vi "Process File.vi"(8 "error in (no error)":errorcluster, 10 "File":path, 11 "NHMFL Synthesizer in":refnum<class "NHMFL Synthesizer.lvclass">) -> (0 "error out":errorcluster, 2 "File out":path, 3 "NHMFL Synthesizer out":refnum<class "NHMFL Synthesizer.lvclass">)   [LabVIEW 2016, in "NHMFL Synthesizer.lvclass"]
uses:
  NHMFL Synthesizer.lvclass
  NHMFL Synthesizer.lvclass/NHMFL Synthesizer.ctl
  Read NHMFL Synthesizer Configuration.vi
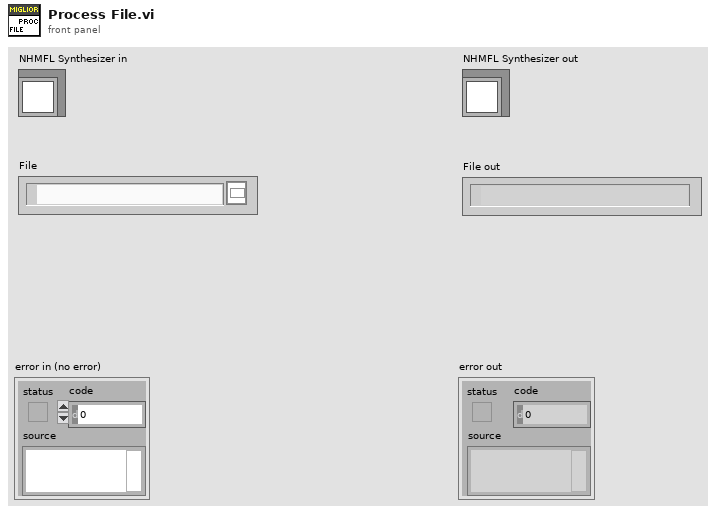
[diagram p1: front panel]
types:
  T1 = enum16{"open", "open or create", "create or replace", "create", "open (read-only)"}
  T2 = typedef "Actual Settings.ctl" = cluster{"Clock/F1":ext, "Clock/F2":ext, "F1":ext, "F2":ext, "Clock":ext}
  T3 = typedef "NHMFL Synthesizer Configuration.ctl" = cluster{"DAQmx Device":tag, "Variable amplitude frequency":dbl, "Fixed amplitude frequency":dbl, "Amplitude":dbl, "Clock multiplier":i32, "Cannel names (variable F)":string[], "Cannel names (fixed F)":string[], "Group":string}
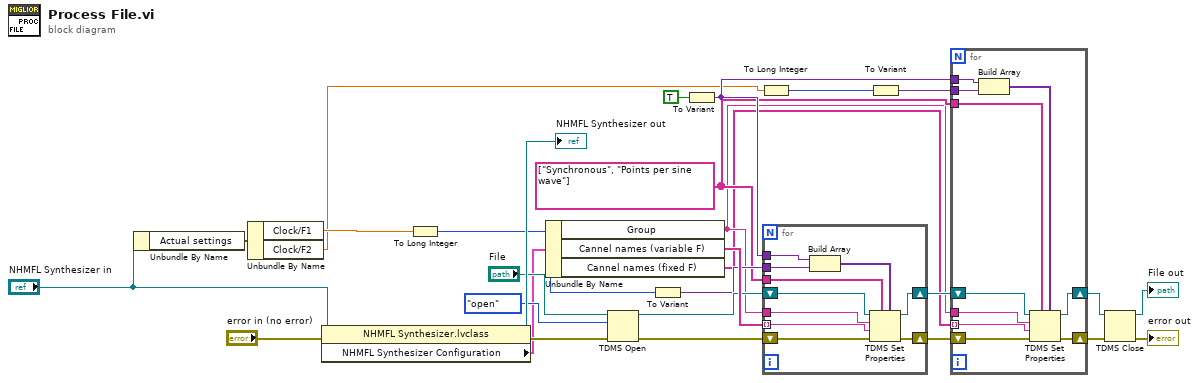
[diagram p0: block diagram]
diagram:
  w7 = string[] ["Synchronous", "Points per sine wave"] ("property names")
  n1 = Unbundle By Name("NHMFL Synthesizer in") -> ("Actual settings"=w18:T2)
  n2 = Unbundle By Name(w18) -> ("Clock/F1"=w16:ext, "Clock/F2"=w10:ext)
  n3 = property class="NHMFL Synthesizer.lvclass"(reference="NHMFL Synthesizer in", error in="error in (no error)") -> (reference out=→"NHMFL Synthesizer out":refnum<class "NHMFL Synthesizer.lvclass">, error out=w24:errorcluster, "NHMFL Synthesizer Configuration"=w22:T3)
  n4 = To Long Integer(number=w16) -> (32bit integer=w15:i32)
  n5 = Unbundle By Name(w22) -> ("Group"=w6:string, "Cannel names (variable F)"=w21:string[], "Cannel names (fixed F)"=w5:string[])
  n6 = TDMS Open(8:w24, 10:T1."open" ("operation (0:open)"), 11:"File") -> (0:w19:errorcluster, 3:w20:refnum<k34>)  [unwired: 4 in]
  n7 = To Variant(anything=w15) -> (Variant=w14:variant)
  n8 = To Variant(anything=TRUE) -> (Variant=w11:variant)
  n9 = To Long Integer(number=w10) -> (32bit integer=w9:i32)
  n10 = for {
    tunnel: w21 -> [w35] mode=indexing
    shift-right: [w33] -> w13
    shift-left: w20 -> [w38]
    shift-right: [w34] -> w12
    shift-left: w19 -> [w37]
    tunnel: w6 -> [w36]
    tunnel: w7 -> [w32]
    tunnel: w11 -> [w31]
    tunnel: w14 -> [w30]
    n11 = Build Array(w31, w30) -> (w29:variant[])
    n12 = TDMS Set Properties(5:w29, 7:w32, 8:w37, 9:w35, 10:w36, 11:w38) -> (0:w34:errorcluster, 3:w33:refnum<k34>)  [unwired: 2 out]
  }
  n13 = To Variant(anything=w9) -> (Variant=w8:variant)
  n14 = for {
    tunnel: w5 -> [w45] mode=indexing
    shift-right: [w43] -> w3
    shift-left: w13 -> [w48]
    shift-right: [w44] -> w4
    shift-left: w12 -> [w47]
    tunnel: w6 -> [w46]
    tunnel: w7 -> [w42]
    tunnel: w11 -> [w41]
    tunnel: w8 -> [w40]
    n15 = Build Array(w41, w40) -> (w39:variant[])
    n16 = TDMS Set Properties(5:w39, 7:w42, 8:w47, 9:w45, 10:w46, 11:w48) -> (0:w44:errorcluster, 3:w43:refnum<k34>)  [unwired: 2 out]
  }
  n17 = TDMS Close(8:w4, 11:w3) -> (0:→"error out":errorcluster, 3:→"File out":path)
